vi "ConfigureInternalClockSynced.vi"(0 "object in":refnum<class "Hamamatsu_simulated.lvclass">, 2 "FramesPerAquisionCycle":i32, 3 "CameraBufferSize":i32, 5 "error in (no error)":errorcluster, 8 "Master pulse Parameters":T1={"Mode"=1, "Source"=1, "Interval"=1.0, "Burst"=0} {"Source" items=["External"=1, "Software"=2]; "Mode" items=["Continuous"=1, "Start"=2, "Burst"=3]}) -> (14 "object out":refnum<class "Hamamatsu_simulated.lvclass">, 19 "error out":errorcluster)   [LabVIEW 2024, in "Hamamatsu_simulated.lvclass"]
uses:
  Hamamatsu_simulated.lvclass
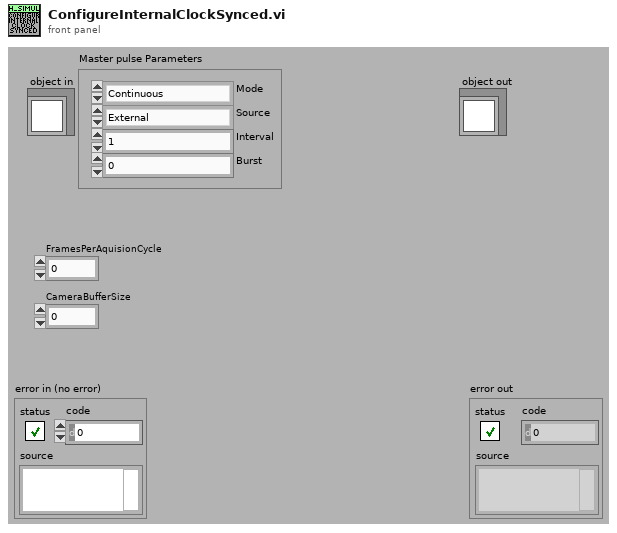
[diagram p1: front panel]
types:
  T1 = cluster{"Mode":u32, "Source":u32, "Interval":dbl, "Burst":u32}
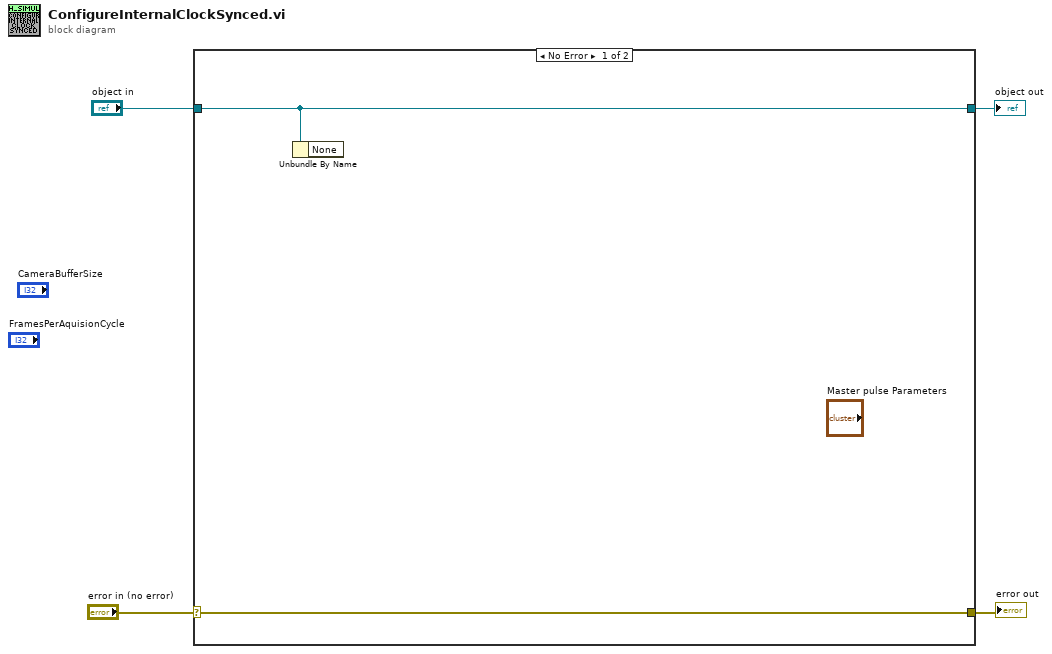
[diagram p0: block diagram]
diagram:
  n1 = case shown="No Error" "error in (no error)" {
    selector: "error in (no error)" -> [w6 w8]
    tunnel: [w6 w8] -> w3
    tunnel: [w5 w7] -> w1
    tunnel: "object in" -> [w5 w7]
    frame No Error {
      n2 = Unbundle By Name(w5) -> ()  [unwired: 1 out]
    }
    frame Error {
    }
  }
  "error out" <- w3
  "object out" <- w1
